vi "AUTOFLIM_Align_Fast.vi"(0 "Z Scan Range":dbl=1.0, 2 "System no.":i32, 5 "Scan Termination":T1(ring), 11 "error in (no error)":errorcluster) -> (3 "Mesh out":dbl, 4 "X Center Out":dbl, 6 "Y Center Out":dbl, 8 "Alignment Graph":dbl[][](array[numeric]), 14 "Z coordinate":dbl, 15 "error out":errorcluster)   [LabVIEW 2023]
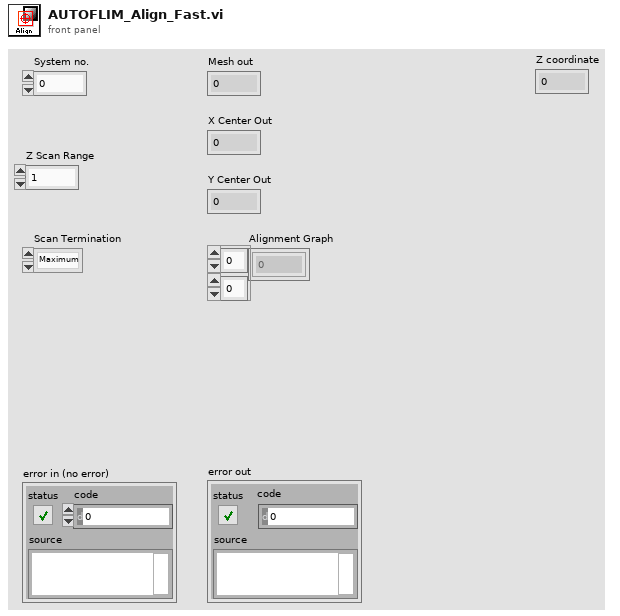
[diagram p1: front panel]
types:
  T1 = enum16{"Maximum", "End Position", "Center of scan"}
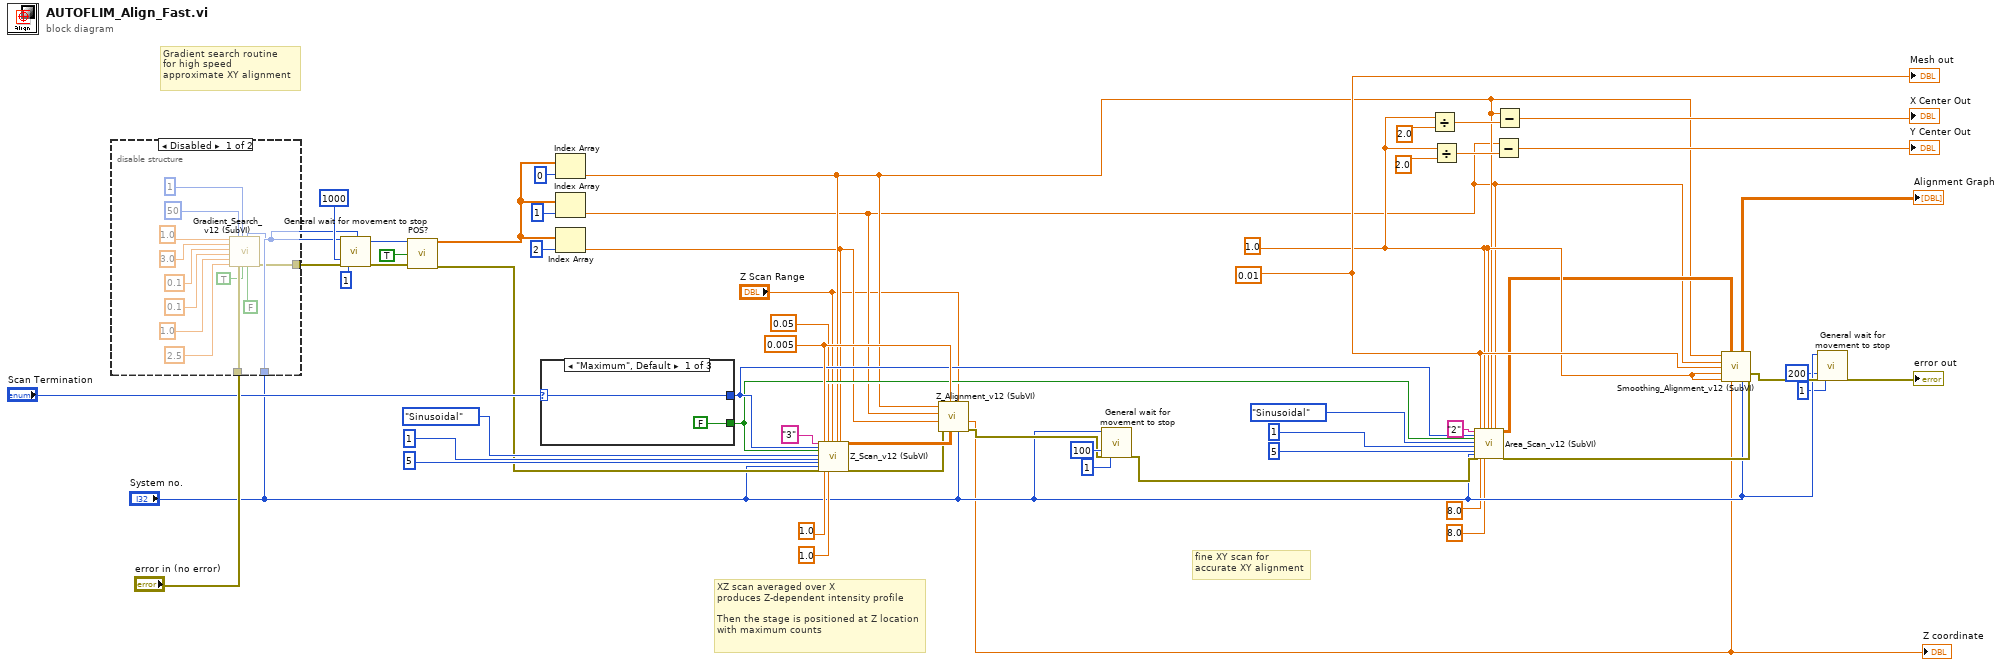
[diagram p0: block diagram]
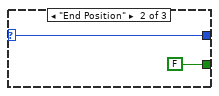
[diagram p3: hidden frame]
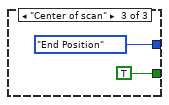
[diagram p4: hidden frame]
diagram:
  w55 = 0.01 ("Mesh in")
  w54 = 1.0 ("X Scan Range")
  w53 = 0.005 ("Z Mesh")
  # "fine XY scan for\naccurate XY alignment"
  # "XZ scan averaged over X\nproduces Z-dependent intensity profile\n\nThen the stage is positioned at Z location\nwith maximum counts"
  # "Gradient search routine\nfor high speed\napproximate XY alignment"
  n1 = disable-structure shown="Disabled" {
    disable-tunnel: "error in (no error)" -> [w59 _]
    disable-tunnel: [w57 _] -> w33
    disable-tunnel: "System no." -> [w56 _]
    frame Disabled {
      n2 = call "Gradient_Search_v12 (SubVI).vi"("Speed factor"=1.0, "Max velocity"=3.0, "ML"=0.1, "Min Radius"=0.1, "Max Radius"=1.0, "GS Frequency"=2.5, "Max. dir. changes"=50, "error in (no error)"=w59, "Analog Input"=1, "Run?"=TRUE, "System no."=w56, "Tracking"=FALSE) -> ("error out"=w57:errorcluster)  [unwired: 7 in]
    }
    frame Enabled {
    }
  }
  n3 = call "General wait for movement to stop.vi"("System no."="System no.", "Additional wait time, ms"=1000, "error in"=w33, "Polling cycle \ntime, ms"=1) -> ("error out"=w25:errorcluster)  [unwired: 4 in, 11 out]
  n4 = call "POS?.vi"("System no."="System no.", "All axes?"=TRUE, "error in"=w25) -> ("Position"=w20:dbl[], "error out"=w23:errorcluster)  [unwired: 2 in, 13 out]
  n5 = case shown="\"Maximum\", Default" "Scan Termination" {
    selector: "Scan Termination" -> [w70 w72 _]
    tunnel: [w70 w72 T1."End Position" ("Scan Termination")] -> w47
    tunnel: [FALSE FALSE TRUE] -> w46
    frame "Maximum", Default {
    }
    frame "End Position" {
    }
    frame "Center of scan" {
    }
  }
  n6 = Index Array(array=w20, index=0) -> (element=w18:dbl)
  n7 = Index Array(array=w20, index=1) -> (element=w17:dbl)
  n8 = Index Array(array=w20, index=2) -> (element=w5:dbl)
  n9 = call "Z_Scan_v12 (SubVI).vi"("Scan Axis"="3", "Scan Termination"=w47, "Center of Scan"=w46, "Scan Type"=enum16{"Sinusoidal", "Spiral"}."Sinusoidal", "Analog Input"=1, "Table rate"=5, "System no."="System no.", "error in (no error)"=w23, "Z Mesh"=w53, "Z-frequency"=1.0, "X Scan Range"=0.05, "Z-velocity"=1.0, "Z Scan Range"="Z Scan Range", "X Scan Center"=w18, "Z Scan Center"=w5) -> ("Intensity Graph"=w28:dbl[][], "error out"=w27:errorcluster)  [unwired: 8 in, 3 out]
  n10 = call "Z_Alignment_v12 (SubVI).vi"("System no."="System no.", "Z range"="Z Scan Range", "Intensity Graph"=w28, "Z Mesh"=w53, "error in (no error)"=w27, "Z"=w5, "Y"=w17, "X"=w18) -> ("error out"=w13:errorcluster, "Zout"=w6:dbl)  [unwired: 2 in]
  "Z coordinate" <- w6
  n11 = call "General wait for movement to stop.vi"("System no."="System no.", "Additional wait time, ms"=u32 100, "error in"=w13, "Polling cycle \ntime, ms"=u32 1 ("Polling cycle \ntime, ms")) -> ("error out"=w12:errorcluster)  [unwired: 4 in, 11 out]
  n12 = Divide(x=w54, y=2.0) -> (x/y=w38:dbl)
  n13 = Divide(x=w54, y=2.0) -> (x/y=w39:dbl)
  n14 = call "Area_Scan_v12 (SubVI).vi"("Step Axis"="2", "Scan Termination"=w47, "Center of Scan"=w46, "Scan Type"=enum16{"Sinusoidal", "Spiral"}."Sinusoidal", "Analog Input"=1, "Table rate"=5, "System no."="System no.", "error in (no error)"=w12, "Mesh in"=w55, "X-frequency"=8.0, "X Scan Range"=w54, "Y-velocity"=8.0 ("X-frequency"), "Y Scan Range"=w54, "X Scan Center"=w18, "Y Scan Center"=w17) -> ("Intensity Graph"=w29:dbl[][], "error out"=w26:errorcluster)  [unwired: 8 in, 3 out]
  n15 = Subtract(x=w17, y=w39) -> (x-y=→"Y Center Out":dbl)
  n16 = Subtract(x=w18, y=w38) -> (x-y=→"X Center Out":dbl)
  n17 = call "Smoothing_Alignment_v12 (SubVI).vi"("X center"=w18, "Intensity Graph"=w29, "Y center"=w17, "Mesh"=w55, "X Scan Range"=w54, "Y Scan Range"=w54, "Z"=w6, "System no."="System no.", "error in (no error)"=w26) -> ("Alignment Graph"=→"Alignment Graph":dbl[][], "error out"=w11:errorcluster)  [unwired: 5 in]
  n18 = call "General wait for movement to stop.vi"("System no."="System no.", "Additional wait time, ms"=u32 200, "error in"=w11, "Polling cycle \ntime, ms"=u32 1 ("Polling cycle \ntime, ms")) -> ("error out"=→"error out":errorcluster)  [unwired: 4 in, 11 out]
  "Mesh out" <- w55
